vi "HAL camera stop.vi"   [LabVIEW 2011]
uses:
  HAL Camera specifications globals.vi
  Camera/camera globals.vi
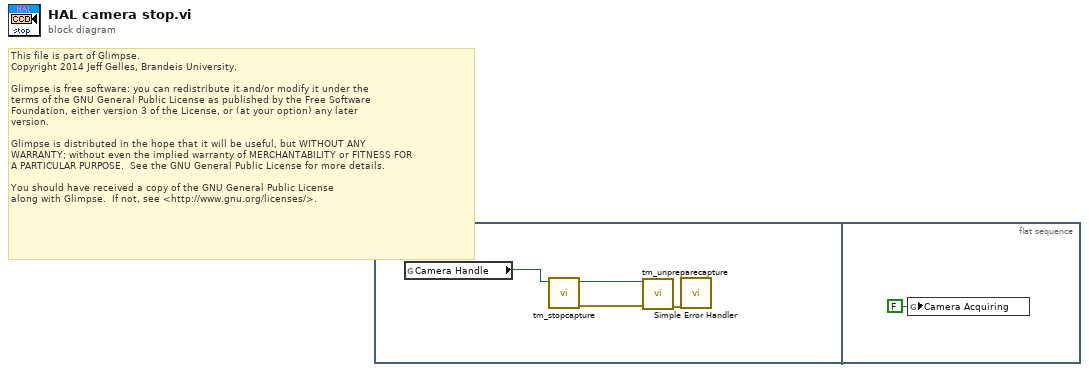
[diagram p0: block diagram]
diagram:
  # "This file is part of Glimpse. \nCopyright 2014 Jeff Gelles, Brandeis University.    \n\nGlimpse is free software: you can redistribute it and/or modify it under the \nterms of the GNU General Public License as published by the Free Software \nFoundation, either version 3 of the License, or (at your option) any later \nversion.\n\nGlimpse is distributed in the hope that it will be useful, but WITHOUT ANY \nWARRANTY; without even the implied warranty of MERCHANTABILITY or FITNESS FOR \nA PARTICULAR PURPOSE.  See the GNU General Public License for more details.\n\nYou should have received a copy of the GNU General Public License\nalong with Glimpse.  If not, see <http://www.gnu.org/licenses/>."
  n1 = flat-sequence {
    frame #0 {
      n2 = global read "HAL Camera specifications globals.vi" "Camera Handle"() -> (w4:u32)
      n3 = call <userlib>:"tm_stopcapture.vi"("Handle in"=w4) -> ("error out"=w3:errorcluster, "Handle out"=w2:u32)  [unwired: 9 in]
      n4 = call <userlib>:"tm_unpreparecapture.vi"("error in (no error)"=w3, "Handle in"=w2) -> ("error out"=w1:errorcluster)  [unwired: 8 in, 1 out]
      n5 = call <vilib>:"Simple Error Handler.vi"("error in (no error)"=w1) -> ()  [unwired: 4 in, 5 out]
    }
    frame #1 {
      n6 = global write "camera globals.vi" "Camera Acquiring"(FALSE ("Andor Aquiring")) -> ()
    }
  }
